vi "std11a.vi"(1 "mean":sgl, 2 "Y":i16[](array[numeric])) -> (0 "std":sgl)   [LabVIEW 2010]
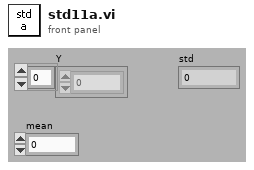
[diagram p1: front panel]
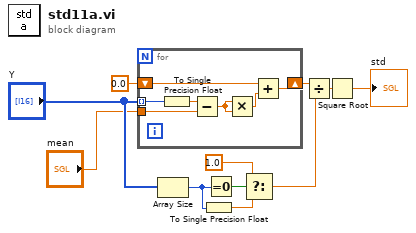
[diagram p0: block diagram]
diagram:
  n1 = for {
    tunnel: "Y" -> [w12] mode=indexing
    tunnel: "mean" -> [w18]
    shift-right: [w14] -> w2
    shift-left: sgl 0.0 -> [w13]
    n2 = To Single Precision Float(number=w12) -> (single precision float=w17:sgl)
    n3 = Subtract(x=w17, y=w18) -> (x-y=w16:sgl)
    n4 = Multiply(x=w16, y=w16) -> (x*y=w15:sgl)
    n5 = Add(x=w13, y=w15) -> (x+y=w14:sgl)
  }
  n6 = Array Size(array="Y") -> (size(s)=w5:i32)
  n7 = To Single Precision Float(number=w5) -> (single precision float=w7:sgl)
  n8 = Equal To 0?(x=w5) -> (x = 0?=w6:bool)
  n9 = Select(t=sgl 1.0, s=w6, f=w7) -> (s? t:f=w9:sgl)
  n10 = Divide(x=w2, y=w9) -> (x/y=w4:sgl)
  n11 = Square Root(x=w4) -> (sqrt(x)=→"std":sgl)
